vi "MotorTester.vi"() -> ()   [LabVIEW 2018]
uses:
  <vilib>/myRIO/Instrument Drivers/Onboard IO/PWM/typedefs/PWM Configuration.ctl
  <vilib>/myRIO/Instrument Drivers/Onboard IO/PWM/PWM.lvlib
  <vilib>/myRIO/Common/Instrument Driver Framework/myRIO v1.0/PWM/typedefs/PWM Channels Enum.ctl
  <vilib>/myRIO/Common/Instrument Driver Framework/Utilities/typedefs/Generic FPGA Reference.ctl
  <vilib>/myRIO/Common/Instrument Driver Framework/Utilities/typedefs/myRIO v1.0 Reference.ctl
  <vilib>/myRIO/Common/Instrument Driver Framework/Utilities/typedefs/Hardware Version Enum.ctl
  <vilib>/myRIO/Common/Instrument Driver Framework/Utilities/typedefs/myRIO Generic Hardware Reference.ctl
  <vilib>/myRIO/Instrument Drivers/Onboard IO/PWM/typedefs/PWM Reference.ctl
  <vilib>/myRIO/Instrument Drivers/Onboard IO/PWM/vis/Set Duty Cycle and Frequency.vi
  <vilib>/userdefined/High Color/nirio_resource_hc.ctl
  <vilib>/myRIO/Common/Instrument Driver Framework/myRIO v1.0/PWM/vis/myRIO v1.1 Open PWM.vi
  <vilib>/myRIO/Instrument Drivers/Onboard IO/PWM/vis/myRIO PWM Open.xnode
  <vilib>/myRIO/Common/Instrument Driver Framework/Utilities/vis/Is FPGA Ref Available.vi
  <vilib>/myRIO/Express VI/Onboard IO/PWM/PWM Express VI.xnode
  <vilib>/myRIO/Common/Instrument Driver Framework/myRIO v1.0/DIO/typedefs/DIO Channels Enum.ctl
  <vilib>/myRIO/Common/Instrument Driver Framework/myRIO v1.0/DIO/typedefs/DIO Channels List.ctl
  <vilib>/myRIO/Instrument Drivers/Onboard IO/DIO/typedefs/DIO Reference.ctl
  <vilib>/myRIO/Instrument Drivers/Onboard IO/DIO/DIO.lvlib
  <vilib>/myRIO/Instrument Drivers/Onboard IO/DIO/vis/Write.vi
  <vilib>/myRIO/Common/Instrument Driver Framework/myRIO v1.0/DIO/vis/myRIO v1.1 Open DIO.vi
  <vilib>/myRIO/Instrument Drivers/Onboard IO/DIO/vis/myRIO DIO Open.xnode
  <vilib>/myRIO/Express VI/Onboard IO/DO/DO Express VI.xnode
  <vilib>/Platform/TimedLoop/XDataNode/XDataNode.xnode
  <vilib>/Platform/TimedLoop/XDataNode/nitl_modes.ctl
  <vilib>/Platform/TimedLoop/XDataNode/XDNodeRunTimeDep.lvlib
  <vilib>/Platform/TimedLoop/XDataNode/wakeup.ctl
  <vilib>/Platform/TimedLoop/XDataNode/timing_clust.ctl
  <vilib>/myRIO/Instrument Drivers/Utilities/Utilities.lvlib
panel:
  in  "Light":dbl=0.4
  out "ENC":T1
  in  "stop":bool
  out "ENC Val. mm":T2
  in  "Encoder PPR":dbl=24.0
  in  "Gear Ratio":i32=64
  in  "R(mm)":dbl=50.0
  in  "Reset Counter":bool
  in  "Motor C":dbl(slide) scale=-100.0..100.0
  in  "Motor B":dbl(slide) scale=-100.0..100.0
  in  "Motor A":dbl(slide) scale=-100.0..100.0
  in  "error in":errorcluster
  out "error out":errorcluster
  in  "Enable":bool
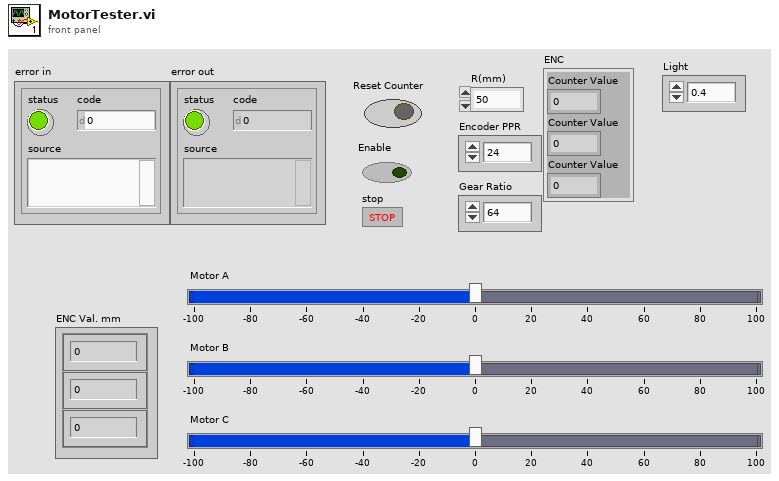
[diagram p1: front panel]
types:
  T1 = cluster{"Counter Value":i32, "Counter Value":i32, "Counter Value":i32}
  T2 = cluster{"Numeric Control":dbl, "Numeric Control":dbl, "Numeric Control":dbl}
  T3 = typedef "XDNodeRunTimeDep.lvlib/timing_clust.ctl" = cluster{"Expected End [f-1]":u64, "Actual End [f-1]":u64, "Finished Late? [f-1]":bool, "Expected End [i-1]":u64, "Actual End [i-1]":u64, "Finished Late? [i-1]":bool, "Expected Start [i]":u64, "Actual Start [i]":u64, "Expected Start [f]":u64, "Actual Start [f]":u64, "Source Name":string, "Structure Name":string, "Period":i64, "Deadline":i64, "Offset":i64, "Start":i64, "Priority":i32, "Timeout":i32, "Mode":T4, "Wakeup Reason":T5, "Error":errorcluster, "Source Type":string, "Secondary Source Type":string, "Global End Time":u64, "Global Start Time":u64, "Frame Duration":u64, "Iteration Duration":u64, "Assigned CPU":i32, "I/O Scan Engine Mode":u32}
  T4 = typedef "XDNodeRunTimeDep.lvlib/nitl_modes.ctl" = enum32{"No Change", "Process missed periods, maintain original phase", "Discard missed periods, maintain original phase", "Process missed periods, ignore original phase", "Discard missed periods, ignore original phase"}
  T5 = typedef "XDNodeRunTimeDep.lvlib/wakeup.ctl" = enum32{"Normal", "Aborted", "Asynchronous wakeup", "Timing source error", "Timed loop error", "Timeout"}
  T6 = typedef "DIO.lvlib/DIO Reference.ctl" = cluster{"myRIO Reference":T7, "DIO Channels List":T11}
  T7 = typedef "myRIO Generic Hardware Reference.ctl" = cluster{"myRIO Model":T8, "myRIO Hardware Reference":T9}
  T8 = typedef "Hardware Version Enum.ctl" = enum16{"Unknown", "myRIO-1900", "myRIO-1950", "roboRIO", "NI ELVIS RIO CM", "ELVIS III"}
  T9 = typedef "myRIO v1.0 Reference.ctl" = cluster{"Generic FPGA Reference":T10, "Allow multiple opens":bool}
  T10 = typedef "Generic FPGA Reference.ctl" = refnum<k20>
  T11 = typedef "DIO Channels List.ctl" = T12[]
  T12 = typedef "DIO Channels Enum.ctl" = enum16{"Not Connected", "C/DIO0", "C/DIO1", "C/DIO2", "C/DIO3", "C/DIO4", "C/DIO5", "C/DIO6", "C/DIO7", "A/DIO0", "A/DIO1", "A/DIO2", "A/DIO3", "A/DIO4", "A/DIO5", "A/DIO6", "A/DIO7", "A/DIO8", "A/DIO9", "A/DIO10", "A/DIO11", "A/DIO12", "A/DIO13", "A/DIO14", "A/DIO15", "A/DIO16", "A/DIO17", "A/DIO18", "A/DIO19", "B/DIO0", "B/DIO1", "B/DIO2", "B/DIO3", "B/DIO4", "B/DIO5", "B/DIO6", "B/DIO7", "B/DIO8", "B/DIO9", "B/DIO10", "B/DIO11", "B/DIO12", "B/DIO13", "B/DIO14", "B/DIO15", "B/DIO16", "B/DIO17", "B/DIO18", "B/DIO19", "LED0", "LED1", "LED2", "LED3", "Button0", "DIO/DIO0", "DIO/DIO1", "DIO/DIO2", "DIO/DIO3", "DIO/DIO4", "DIO/DIO5", "DIO/DIO6", "DIO/DIO7", "DIO/DIO8", "DIO/DIO9", "SPI/CS0", "SPI/CS1", "SPI/CS2", "SPI/CS3", "LED RADIO (Green)", "LED RADIO (Red)", "LED COMM (Green)", "LED COMM (Red)", "LED MODE (Green)", "LED MODE (Red)"}
  T13 = typedef "nirio_resource_hc.ctl" = tag
  T14 = typedef "PWM.lvlib/PWM Reference.ctl" = cluster{"myRIO Reference":T7, "PWM Channels Enum":T15, "PWM Configuration":T16}
  T15 = typedef "PWM Channels Enum.ctl" = enum16{"Not Connected", "C/PWM0", "C/PWM1", "A/PWM0", "A/PWM1", "A/PWM2", "A/PWM3", "A/PWM4", "A/PWM5", "A/PWM6", "A/PWM7", "A/PWM8", "A/PWM9", "A/PWM10", "A/PWM11", "A/PWM12", "A/PWM13", "A/PWM14", "A/PWM15", "A/PWM16", "A/PWM17", "A/PWM18", "A/PWM19", "B/PWM0", "B/PWM1", "B/PWM2", "B/PWM3", "B/PWM4", "B/PWM5", "B/PWM6", "B/PWM7", "B/PWM8", "B/PWM9", "B/PWM10", "B/PWM11", "B/PWM12", "B/PWM13", "B/PWM14", "B/PWM15", "B/PWM16", "B/PWM17", "B/PWM18", "B/PWM19", "PWM/PWM0", "PWM/PWM1", "PWM/PWM2", "PWM/PWM3", "PWM/PWM4", "PWM/PWM5", "PWM/PWM6", "PWM/PWM7", "PWM/PWM8", "PWM/PWM9"}
  T16 = typedef "PWM.lvlib/PWM Configuration.ctl" = cluster{"Frequency":dbl, "Duty Cycle":dbl}
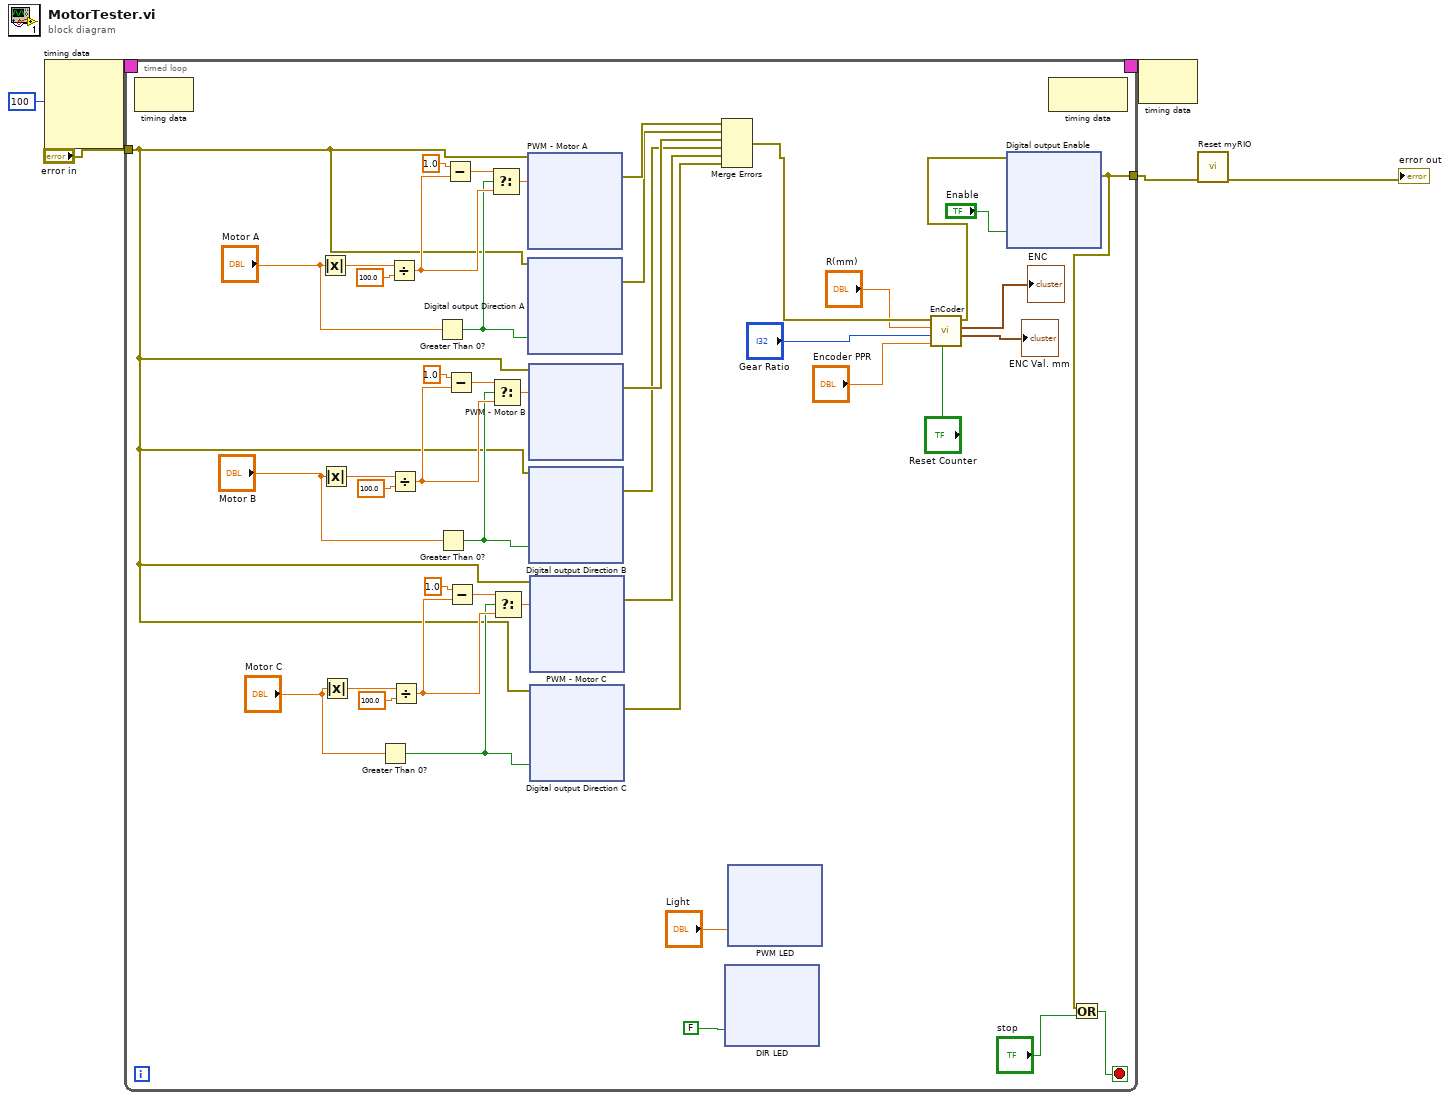
[diagram p0: block diagram]
diagram:
  n1 = node-c288(i64 100 ("Period")) -> (w5:T3)  [unwired: 3 in]
  n2 = timed-loop {
    tunnel: [w10] -> w2
    tunnel: "error in" -> [w13]
    timing: w5 -> [_]
    timing-out: [_] -> w4
    stop <- w9 stop-if-true
    n3 = node-c288() -> ()  [unwired: 1 in, 1 out]
    n4 = Absolute Value(x="Motor A") -> (abs(x)=w47:dbl)
    n5 = Absolute Value(x="Motor B") -> (abs(x)=w39:dbl)
    n6 = Absolute Value(x="Motor C") -> (abs(x)=w34:dbl)
    n7 = Greater Than 0?(x="Motor C") -> (x > 0?=w28:bool)
    n8 = Divide(x=w47, y=100.0) -> (x/y=w44:dbl)
    n9 = Divide(x=w39, y=100.0) -> (x/y=w41:dbl)
    n10 = Divide(x=w34, y=100.0) -> (x/y=w32:dbl)
    n11 = Greater Than 0?(x="Motor A") -> (x > 0?=w30:bool)
    n12 = Greater Than 0?(x="Motor B") -> (x > 0?=w29:bool)
    n13 = Subtract(x=1.0, y=w44) -> (x-y=w43:dbl)
    n14 = Subtract(x=1.0, y=w41) -> (x-y=w42:dbl)
    n15 = Subtract(x=1.0, y=w32) -> (x-y=w31:dbl)
    n16 = Select(t=w43, s=w30, f=w44) -> (s? t:f=w48:dbl)
    n17 = Select(t=w42, s=w29, f=w41) -> (s? t:f=w38:dbl)
    n18 = Select(t=w31, s=w28, f=w32) -> (s? t:f=w35:dbl)
    n19 = xnode "PWM - Motor A"("Duty Cycle"=w48, "error in (no error)"=w13) -> ("error out"=w51:errorcluster)
    n20 = xnode "Digital output Direction A"("DIRA (A/DIO13 (Pin 26))"=w30, "error in (no error)"=w13) -> ("error out"=w50:errorcluster)
    n21 = xnode "PWM - Motor B"("Duty Cycle"=w38, "error in (no error)"=w13) -> ("error out"=w27:errorcluster)
    n22 = xnode "Digital output Direction B"("DIRB (B/DIO13 (Pin 26))"=w29, "error in (no error)"=w13) -> ("error out"=w26:errorcluster)
    n23 = xnode "PWM - Motor C"("Duty Cycle"=w35, "error in (no error)"=w13) -> ("error out"=w25:errorcluster)
    n24 = xnode "Digital output Direction C"("DIRC (C/DIO1 (DIO1))"=w28, "error in (no error)"=w13) -> ("error out"=w24:errorcluster)
    n25 = Merge Errors(w51, w50, w27, w26, w25, w24) -> (w19:errorcluster)
    n26 = xnode "DIR LED"("DIRC (C/DIO5 (DIO5))"=FALSE) -> ()  [unwired: 1 in, 1 out]
    n27 = xnode "PWM LED"("Duty Cycle"="Light") -> ()  [unwired: 1 in, 1 out]
    n28 = call "EnCoder.vi"("Reset Counter"="Reset Counter", "Encoder PPR"="Encoder PPR", "Gear Ratio"="Gear Ratio", "R(mm)"="R(mm)", "error in"=w19) -> ("ENC Val. mm"=→"ENC Val. mm":T2, "ENC"=→"ENC":T1, "error out"=w18:errorcluster)  [unwired: 4 in]
    n29 = xnode "Digital output Enable"("ENABLE (A/DIO4 (Pin 19))"="Enable", "error in (no error)"=w18) -> ("error out"=w10:errorcluster)
    n30 = node-c288() -> ()  [unwired: 1 in, 1 out]
    n31 = Or(x=w10, y="stop") -> (x .or. y?=w9:bool)
  }
  n32 = node-c288(w4) -> ()  [unwired: 1 out]
  n33 = call <vilib>:"Reset myRIO.vi"("error in (no error)"=w2) -> ("error out"=→"error out":errorcluster)  [unwired: 10 in]
